vi "Check Output Message Frame Type.vi"(7 "Data to Send":T2 {"Identifier" format="%08x"}) -> (8 "Frame Type":T1)   [LabVIEW 2013, in "J1939.lvlib"]
uses:
  J1939.lvlib
  API Types/CAN Outgoing Message Cluster.ctl
  API Types/Outgoing Messages Frame Type.ctl
  Frame Conversion/Convert CAN Arb ID to J1939 ID.vi
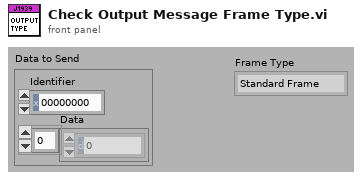
[diagram p1: front panel]
types:
  T1 = typedef "J1939.lvlib/Outgoing Messages Frame Type.ctl" = enum16{"Standard Frame", "BAM", "Connection Mode"}
  T2 = typedef "J1939.lvlib/CAN Outgoing Message Cluster.ctl" = cluster{"Identifier":u32, "Data":u8[]}
  T3 = typedef "J1939.lvlib/PGN Fields Cluster.ctl" = cluster{"Reserved Bit":u8, "Data page":u8, "PDU Format":u8, "PDU Specific":u8}
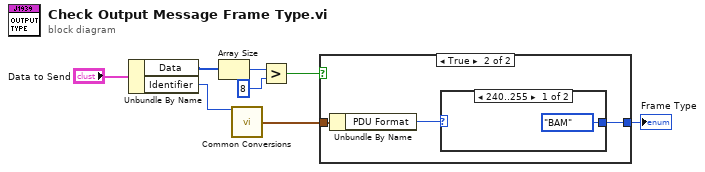
[diagram p0: block diagram]
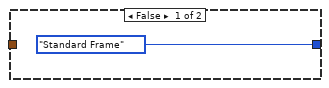
[diagram p2: hidden frame]
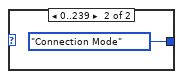
[diagram p3: hidden frame]
diagram:
  n1 = Unbundle By Name("Data to Send") -> ("Data"=w6:u8[], "Identifier"=w3:u32)
  n2 = Array Size(array=w6) -> (size(s)=w7:i32)
  n3 = call-poly "Common Conversions.vi"("Arb ID"=w3) -> ("PGN Fields"=w2:T3)  [unwired: 14 out]
  n4 = Greater?(x=w7, y=8) -> (0:w4:bool)
  n5 = case shown="True" w4 {
    tunnel: [Outgoing_Messages_Frame_Type."Standard Frame" ("Enum") w10] -> w1
    tunnel: w2 -> [_ w12]
    frame False {
    }
    frame True {
      n6 = Unbundle By Name(w12) -> ("PDU Format"=w11:u8)
      n7 = case shown="240..255" w11 {
        tunnel: [Outgoing_Messages_Frame_Type."BAM" ("Enum") Outgoing_Messages_Frame_Type."Connection Mode" ("Enum")] -> w10
        frame 240..255 {
        }
        frame 0..239 {
        }
      }
    }
  }
  "Frame Type" <- w1
